vi "P3Y1.vi"() -> ()   [LabVIEW 2020]
uses:
  <vilib>/Utility/error.llb/DialogType.ctl
panel:
  out "x/y":dbl
  in  "Y":dbl
  in  "X":dbl
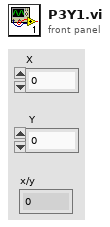
[diagram p1: front panel]
types:
  T1 = typedef "DialogType.ctl" = u16
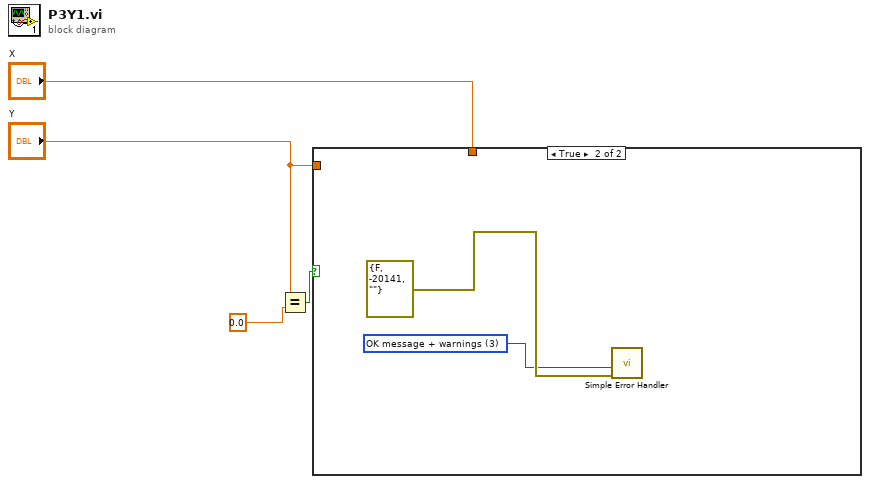
[diagram p0: block diagram]
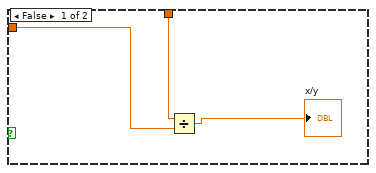
[diagram p2: hidden frame]
diagram:
  n1 = Equal?(x="Y", y=0.0) -> (x = y?=w3:bool)
  n2 = case shown="True" w3 {
    tunnel: "X" -> [w7 _]
    tunnel: "Y" -> [w6 _]
    frame False {
      n3 = Divide(x=w7, y=w6) -> (x/y=→"x/y":dbl)
    }
    frame True {
      w8 = T1 3 items=["no dialog", "OK message", "continue or stop message", "OK message + warnings", "continue/stop + warnings"] ("type of dialog (OK msg:1)")
      n4 = call <vilib>:"Simple Error Handler.vi"("type of dialog (OK msg:1)"=w8, "error in (no error)"=errorcluster {"status"=FALSE, "code"=-20141, "source"=""} ("error constant")) -> ()  [unwired: 3 in, 5 out]
    }
  }
